vi "Shutdown.vi"(8 "error in":errorcluster, 11 "PIOD in":refnum<class "PIOD.lvclass">) -> (0 "error out":errorcluster, 3 "PIOD out":refnum<class "PIOD.lvclass">)   [LabVIEW 2018, in "PIOD.lvlib" / "PIOD.lvclass"]
uses:
  PIOD.lvclass
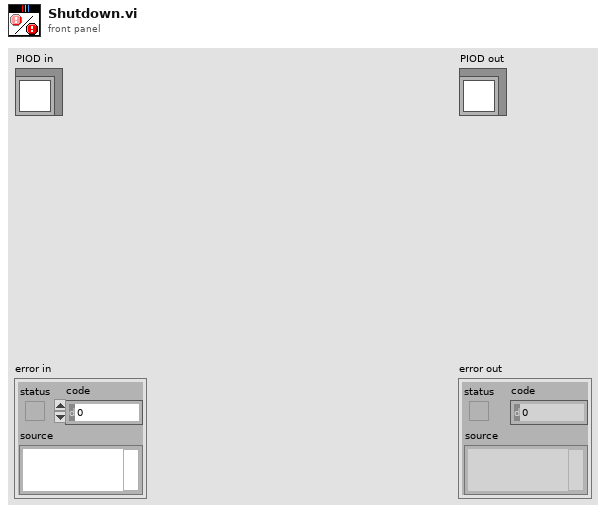
[diagram p1: front panel]
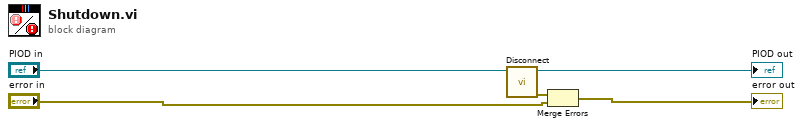
[diagram p0: block diagram]
diagram:
  n1 = call "Disconnect.vi"("PIOD in"="PIOD in") -> ("error out"=w3:errorcluster, "PIOD out"=→"PIOD out":refnum<class "PIOD.lvclass">)  [unwired: 9 in]
  n2 = Merge Errors(w3, "error in") -> (→"error out":errorcluster)
